vi "OP600ZP_NouveauDossier.vi"(8 "entrée d'erreur (pas d'erreur)":errorcluster, 10 "Nom du repertoire (PN SN)":string, 11 "Network before adding a new folder":path) -> (0 "sortie d'erreur":errorcluster, 3 "Network after adding a new folder":path)   [LabVIEW 2020]
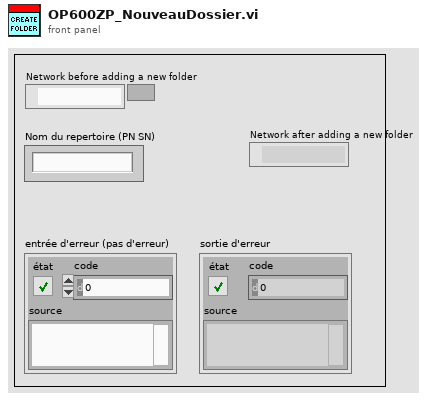
[diagram p1: front panel]
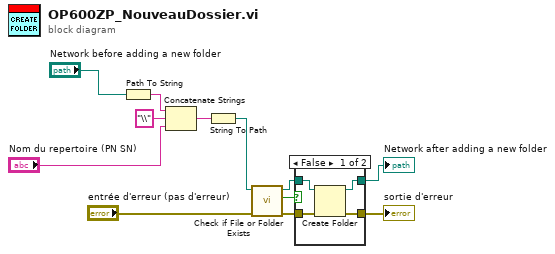
[diagram p0: block diagram]
diagram:
  n1 = Path To String(path="Network before adding a new folder") -> (string=w1:string)
  n2 = Concatenate Strings(w1, "\\" ("chaîne"), "Nom du repertoire (PN SN)") -> (w2:string)
  n3 = String To Path(string=w2) -> (path=w4:path)
  n4 = call <vilib>:"Check if File or Folder Exists.vi"("error in (no error)"="entrée d'erreur (pas d'erreur)", "path"=w4) -> ("error out"=w6:errorcluster, "file or folder exists?"=w9:bool, "dup path"=w7:path)  [unwired: 7 in]
  n5 = case shown="False" w9 {
    tunnel: w6 -> [w16 w18]
    tunnel: w7 -> [w15 w17]
    tunnel: [w14 w18] -> w8
    tunnel: [w13 w17] -> w11
    frame False {
      n6 = Create Folder(path (use dialog)=w15, error in=w16) -> (created path=w13:path, error out=w14:errorcluster)  [unwired: 1 in, 1 out]
    }
    frame True {
    }
  }
  "Network after adding a new folder" <- w11
  "sortie d'erreur" <- w8
